vi "Translation2d_GetNorm.vi"(11 "In Translation":T1 {"Y" format="%14.3f"; "X" format="%14.3f"}) -> (3 "Norm":dbl)   [LabVIEW 2019, in "Trajectory_Library.lvlib"]
doc: "Returns the norm, or distance from the origin to the translation.\n\nParameters:\n - IN TRANSLATION - This translation data structure\n\nReturns:\n - Norm - The norm of the translation."
uses:
  Trajectory_Library.lvlib
  TypeDef/TRANSLATION2D.ctl
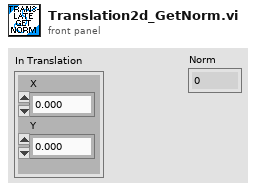
[diagram p1: front panel]
types:
  T1 = typedef "Trajectory_Library.lvlib/TRANSLATION2D.ctl" = cluster{"X":dbl, "Y":dbl}
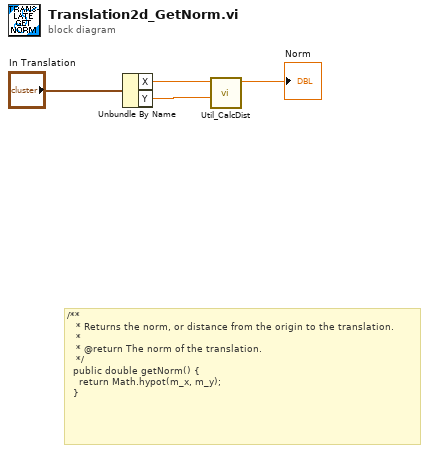
[diagram p0: block diagram]
diagram:
  # "/**\n   * Returns the norm, or distance from the origin to the translation.\n   *\n   * @return The norm of the translation.\n   */\n  public double getNorm() {\n    return Math.hypot(m_x, m_y);\n  }"
  n1 = Unbundle By Name("In Translation") -> ("X"=w2:dbl, "Y"=w1:dbl)
  n2 = call "Util_CalcDist.vi"("Y"=w1, "X"=w2) -> ("DIST"=→"Norm":dbl)  [unwired: 9 in]
